vi "Configure Aux Ouput.vi"(8 "error in (no error)":errorcluster, 9 "Aux Output Voltage (1 V)":dbl=1.0, 10 "Aux Channel (1: Channel 1)":u16(ring)=1 items=["Channel 1"=1, "Channel 2"=2, "Channel 3"=3, "Channel 4"=4], 11 "VISA resource name":refnum<visa-resource-name>) -> (0 "error out":errorcluster, 3 "VISA resource name out":refnum<visa-resource-name>)   [LabVIEW 2017, in "Stanford Research 830.lvlib"]
doc: "Configures the voltage of the aux output channel on the rear panel of the instrument."
uses:
  Users/Biorgel/Documents/Data/Chunxiong Bao/Capacitance/SR830/Stanford Research 830/Stanford Research 830.lvlib
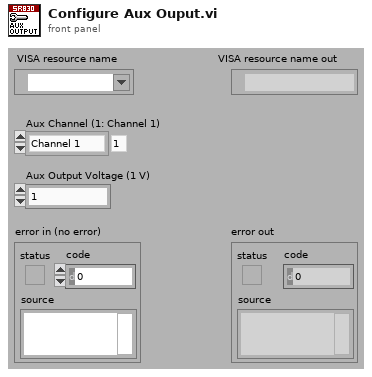
[diagram p1: front panel]
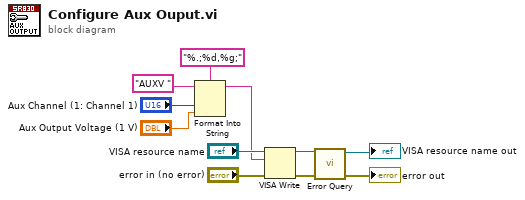
[diagram p0: block diagram]
diagram:
  n1 = Format Into String(format string="%.;%d,%g;", initial string="AUXV ", "Aux Channel (1: Channel 1)", "Aux Output Voltage (1 V)") -> (resulting string=w5:string)  [unwired: 1 in, 1 out]
  n2 = VISA Write(VISA resource name="VISA resource name", write buffer=w5, error in (no error)="error in (no error)") -> (VISA resource name out=w4:refnum<visa-resource-name>, error out=w3:errorcluster)  [unwired: 1 out]
  n3 = call "Error Query.vi"("error in (no error)"=w3, "VISA resource name"=w4) -> ("error out"=→"error out":errorcluster, "VISA resource name out"=→"VISA resource name out":refnum<visa-resource-name>)  [unwired: 7 in, 1 out]
